vi "Tell.vi"(4 "Unified Actor Alias":string, 6 "Unified Actor Relation":T1, 7 "Actor in":refnum<class "Actor.lvclass">, 9 "Msg DVR":refnum<data-value>, 10 "Transport":refnum<user-event>) -> (0 "Error out":errorcluster, 5 "Actor out":refnum<class "Actor.lvclass">)   [LabVIEW 2020, in "jettl.lvlib"]
uses:
  jettl.lvlib
  Actor/Actor.lvclass
  Unified Actor Relation.ctl
  Teller.ctl
  Msg Contents/Msg Contents.lvclass
  Msg.ctl
  Msg/Msg.lvclass
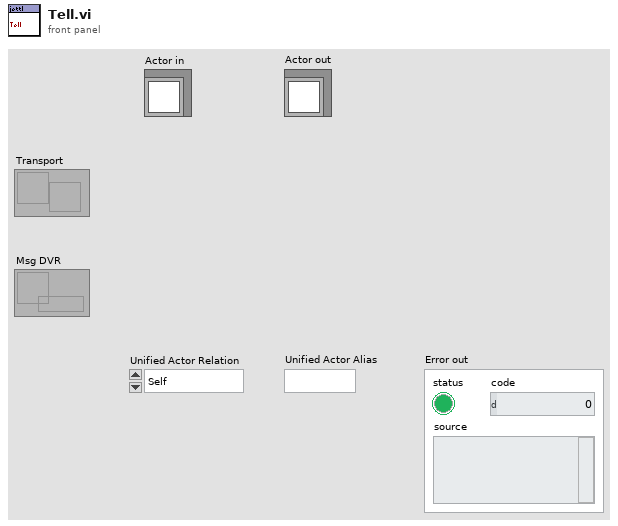
[diagram p1: front panel]
types:
  T1 = typedef "jettl.lvlib/Unified Actor Relation.ctl" = enum16{"Self", "Parent", "Child"}
  T2 = typedef "jettl.lvlib/Msg.ctl" = cluster{"Msg":refnum<class "Msg.lvclass">, "Msg Contents":refnum<class "Msg Contents.lvclass">, "Teller":T3}
  T3 = typedef "jettl.lvlib/Teller.ctl" = cluster{"Unified Actor Alias":string, "Unified Actor Relation":T1, "Absolute Time":timestamp, "Relative Time":dbl}
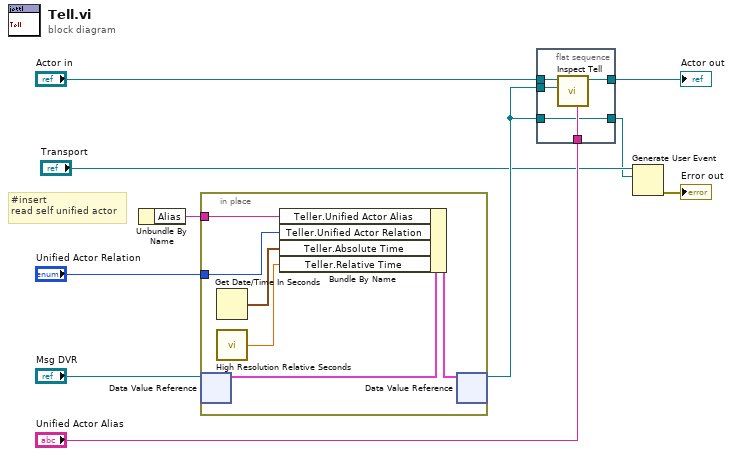
[diagram p0: block diagram]
diagram:
  # "#insert\nread self unified actor"
  n1 = Unbundle By Name() -> ("Alias"=w1:string)  [unwired: 1 in]
  n2 = in-place {
    in-place-border: "Unified Actor Relation" -> [w16]
    in-place-border: w1 -> [w15]
    n3 = in-place-dvr #1("Msg DVR") -> (w14:T2)  [unwired: 1 out]
    n4 = Get Date/Time In Seconds() -> (seconds since 1Jan1904=w11:timestamp)
    n5 = call <vilib>:"High Resolution Relative Seconds.vi"() -> ("relative seconds"=w12:dbl)
    n6 = Bundle By Name(cluster=w14, "Teller.Unified Actor Alias"=w15, "Teller.Unified Actor Relation"=w16, "Teller.Absolute Time"=w11, "Teller.Relative Time"=w12) -> (w13:T2)
    n7 = in-place-dvr #1(w13) -> (w5:refnum<data-value>)  [unwired: 1 out]
  }
  n8 = flat-sequence {
    tunnel: "Unified Actor Alias" -> [w21]
    tunnel: "Actor in" -> [w20]
    tunnel: [w19] -> w7
    tunnel: w5 -> [w18]
    tunnel: [w17] -> w3
    tunnel: w5 -> [w17]
    frame #0 {
      n9 = call-dynamic "Inspect Tell.vi"("Unified Actor Alias"=w21, "Msg DVR"=w18, "Actor in"=w20) -> ("Actor out"=w19:refnum<class "Actor.lvclass">)  [unwired: 8 in]
    }
  }
  n10 = Generate User Event(user event="Transport", event data cluster=w3) -> (error out=→"Error out":errorcluster)  [unwired: 2 in, 1 out]
  "Actor out" <- w7
